vi "Coordinate Space_Setting_UI.vi"(9 "RootPath":path, 10 "Project Name":string, 11 "Image In":T1(plugin-control)) -> (3 "Origin Set":bool)   [LabVIEW 2019]
uses:
  Control/CoordinateUI.ctl
  Control/CoordinateAction.ctl
  Control/DataTransform.ctl
  Process/Controls/Process_Setting.ctl
  Analysis/Controls/Analysis_Setting.ctl
  Controls/Vision_DataEntry.ctl
  Caliper/Controls/Caliper_Entry_FGV_Action.ctl
  Caliper/Controls/AnalysisResultPointsAction.ctl
  Caliper/Controls/CaliperType.ctl
  Caliper/Controls/SelectionListEntryPointType.ctl
  Caliper/Controls/SelectionListEntry.ctl
  Control/CoordinateCaliperSetting.ctl
  Caliper/Controls/CaliperResult.ctl
  Caliper/Controls/CaliperDataEntry.ctl
  <vilib>/Utility/miscctls.llb/LVRowAndColumnTypeDef.ctl
  Analysis/Controls/V_Analysis_Type.ctl
  Ctrl/VisionProcessName.ctl
  Control/CoordinateAnalysisFunc.ctl
panel:
  in  "Done":bool
  out "Numeric":i32
  out "x-y":u32
  out "TempImage":T1(plugin-control)
  in  "Available Points":i32(listbox)=5
  in  "Function_Tab":enum32{"Process", "Analysis", "Caliper"}(tab)
  out "Process Steps":i32(listbox)
  in  "ConfigProcess":bool
  in  "ConfigAnalysis Modify":bool caption="Modify"
  in  "Analysis Delete":bool caption="Delete"
  in  "Analysis Step":i32[](listbox)
  in  "ConfigAnalysis":bool
  in  "Analysis Function":T2
  in  "Caliper Step":i32[](listbox)
  in  "Set Caliper":bool
  in  "Run Test":bool
  in  "CoordExit":bool caption="Exit"
  in  "Set Original":bool
  out "Vision_Image":T1(plugin-control)
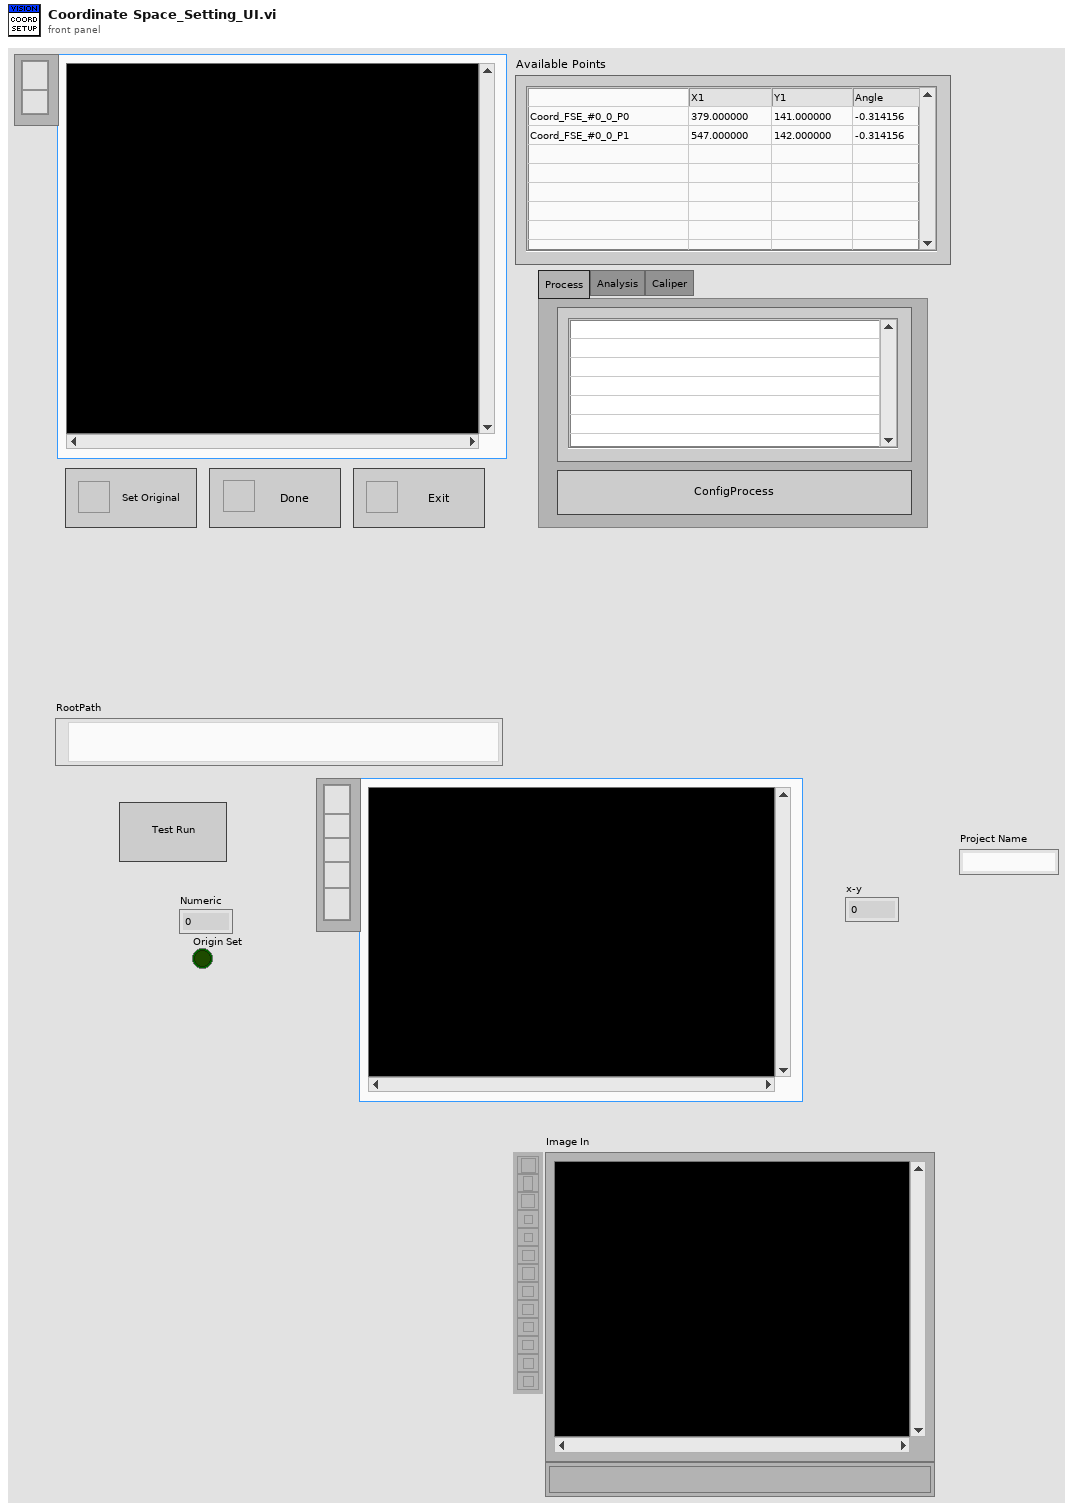
[diagram p1: front panel]
types:
  T1 = typedef "IMAQ Image.ctl" = refnum<image>
  T2 = typedef "CoordinateAnalysisFunc.ctl" = enum16{"Pattern Match", "Find Straight Edge"}
  T3 = typedef "CoordinateUI.ctl" = cluster{"CoordinateUICmd":enum16{"Initialize", "ConfigProcess", "AddAnalysis", "EditAnalysis", "SingleRunWithoutCaliper", "UpdateCaliper", "Run Test", "DeleteAnalysis", "SetOrigin", "UIUpdate", "Done", "Stop", "OriginUpdate", "UpdateOriginList", "Init Read Template"}, "CoordiUIParam":variant}
  T4 = typedef "Image Type" = u32
  T5 = typedef "CoordinateAction.ctl" = enum16{"Initialize", "CoordEntryInput", "CoordEntryOutput", "CoordEntryTemp", "CoordEntryBackup", "CoordEntryReturn"}
  T6 = typedef "LVRowAndColumnTypeDef.ctl" = cluster{"Row":i32, "Column":i32}
  T7 = typedef "Caliper_Entry_FGV_Action.ctl" = enum16{"Init", "Close", "Add", "Delete", "ReplaceAll", "ReadAll"}
  T8 = typedef "Vision_DataEntry.ctl" = cluster{"vROIName":string, "vROIContour":cluster{"Contour Type":u32, "ROI Type":u32, "Points":i32[]}, "ProcessSetting":T9[], "Analysis_Setting":T11}
  T9 = typedef "Process_Setting.ctl" = cluster{"Enum_PreProcess":T10, "Parameter":string}
  T10 = typedef "VisionProcessName.ctl" = enum16{"*CamParameter*", "CamAttributes", "*Preprocess*", "CG_Brightness", "C_Plane Extraction", "C_Threshold", "G_Lookup Table", "G_Threshold"}
  T11 = typedef "Analysis_Setting.ctl" = cluster{"PreProcess":T12, "Parameter":string}
  T12 = typedef "V_Analysis_Type.ctl" = enum16{"None", "C_Color Pattern Matching", "G_PatternMatching", "G_ShapeDectect", "G_GeometricMatch", "B_Area Check"}
  T13 = typedef "DataTransform.ctl" = enum16{"CoordToMain", "MainToCoord"}
  T14 = typedef "CoordinateCaliperSetting.ctl" = cluster{"Result":variant, "CoordinateUse":bool, "CaliperEntry":T15}
  T15 = typedef "CaliperDataEntry.ctl" = cluster{"CaliperType":T16, "Points":T17[], "Result":T19, "StepName":string}
  T16 = typedef "CaliperType.ctl" = u32
  T17 = typedef "SelectionListEntry.ctl" = cluster{"Type":T18, "Index":i32}
  T18 = typedef "SelectionListEntryPointType.ctl" = enum16{"AnalysisResult", "CaliperResult"}
  T19 = typedef "CaliperResult.ctl" = cluster{"PointInclude?":bool, "Num_Of_Pts":u8, "Position.X":dbl, "Position.Y":dbl, "Angle":dbl, "Distance":dbl, "Area":dbl, "Radius_MAX":dbl, "Radius2_min":dbl, "Dev_Residual":dbl, "P2.X":dbl, "P2.Y":dbl, "StepName":string, "Point ID":u8, "StepError?":bool, "ResultDiff?":bool}
  T20 = typedef "AnalysisResultPointsAction.ctl" = enum16{"Init", "Add", "Delete", "ReplaceAll", "ReadAll", "Close"}
  T21 = enum16{"Initialize", "ConfigProcess", "AddAnalysis", "EditAnalysis", "SingleRunWithoutCaliper", "UpdateCaliper", "Run Test", "DeleteAnalysis", "SetOrigin", "UIUpdate", "Done", "Stop", "OriginUpdate", "UpdateOriginList", "Init Read Template"}
  T22 = typedef "CoordinatteEntry.ctl" = cluster{"ProcessSetting":T9[], "Project Name":string, "AnalysisSetting":T23[], "Coord?":bool, "OriginPointInfo":cluster{"Output Original":bool, "Origin Name":string, "Angle":dbl, "Mode":u16, "OriginPoint":cluster{"X":dbl, "Y":dbl}}, "CaliperSetting":T14[], "CoordIndex":i32[]}
  T23 = typedef "CoordinateAnalysisSetting.ctl" = cluster{"Analysis_Type":enum16{"PatternMatch", "Straight Edge"}, "ROI ":T24, "Parameter":variant, "Step Result":variant, "AnalysisStepName":string, "CoordinateUse":bool}
  T24 = typedef "ROI Descriptor" = cluster{"Global Rectangle":i32[], "Contours":cluster{"ID":enum32{"External", "Internal"}, "Type":u32, "Coordinates":i32[]}[]}
  T25 = typedef "Analysis_Setting.ctl" = cluster{"PreProcess":T26, "Parameter":string}
  T26 = typedef "V_Analysis_Type.ctl" = enum16{"None", "C_Color Pattern Matching", "G_PatternMatching"}
  T27 = typedef "Analysis_Setting.ctl" = cluster{"PreProcess":T28, "Parameter":string}
  T28 = typedef "VisionProcessName.ctl" = enum16{"*CamParameter*", "CamAttributes", "*Preprocess*", "CG_Brightness", "C_Plane Extraction", "C_Threshold", "G_Lookup Table", "G_Threshold", "B_Image Inversion", "*Algorithm*", "CG_Histogram", "C_Color Matching", "C_Color Pattern Matching", "G_PatternMatch", "CG_Find Straight Edge", "CG_Adv. Find Straight Edge", "CG_Find Circular Edge", "G_Max Clamp", "G_Clamp (Rake)", "G_Pattern Matching"}
  T29 = typedef "Analysis_Result_To_Caliper.ctl" = cluster{"PointName":string, "Position_X":dbl, "Position_Y":dbl}
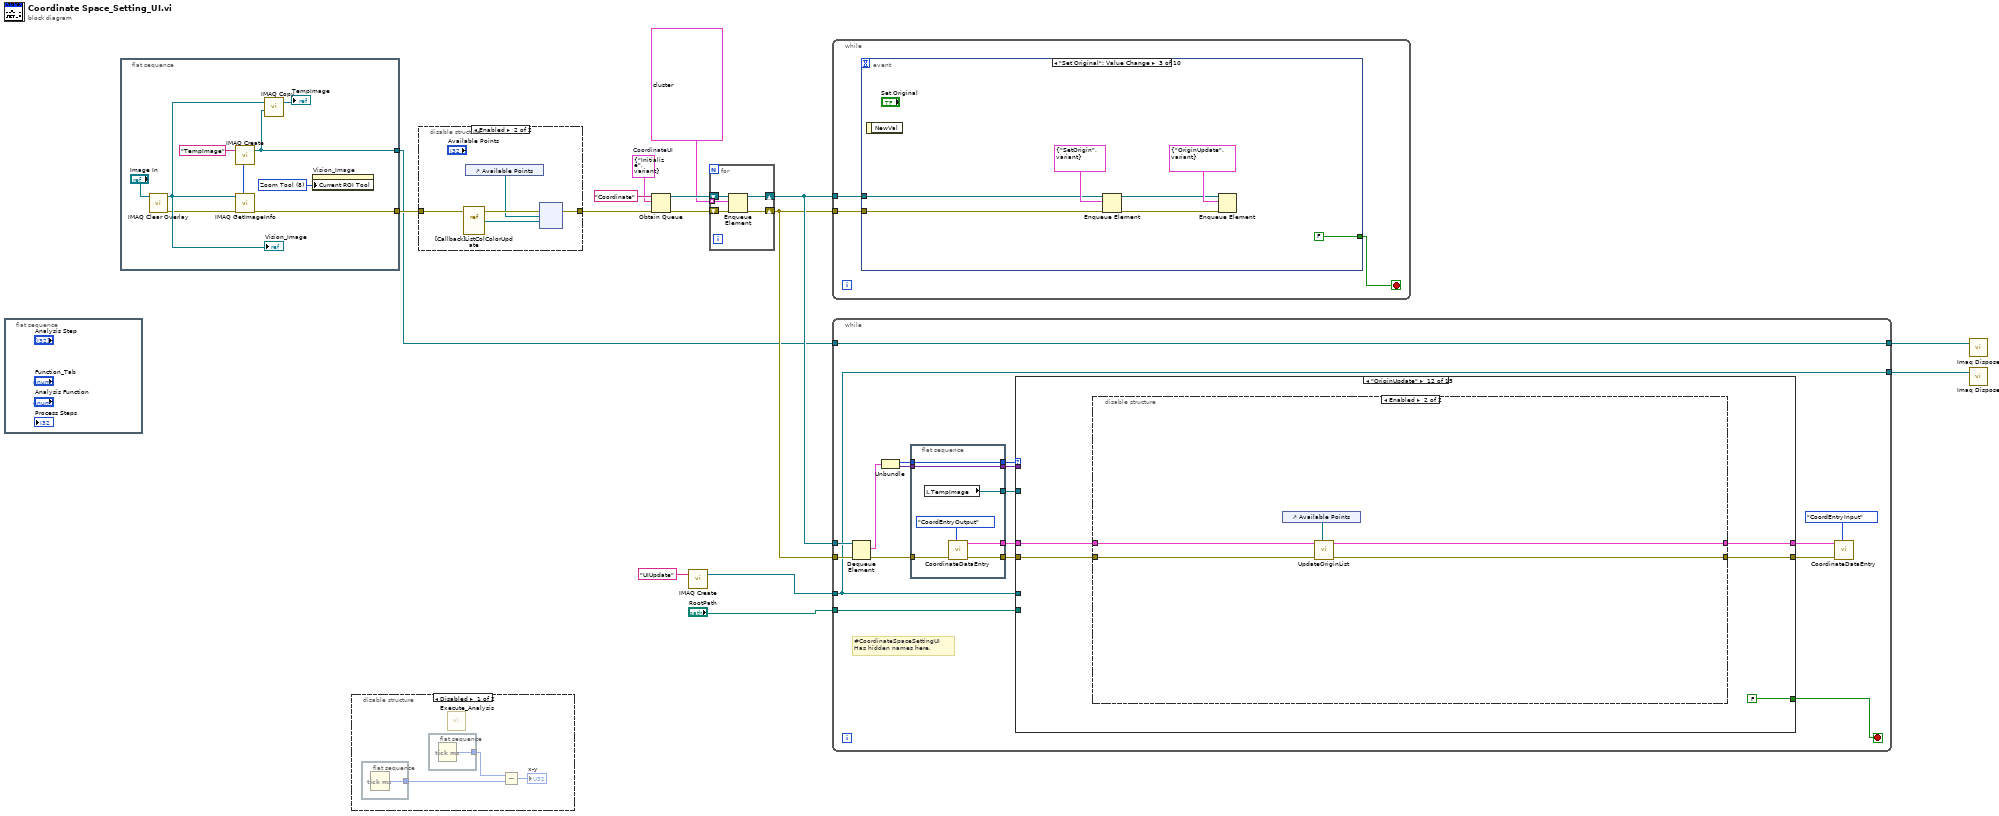
[diagram p0: block diagram]
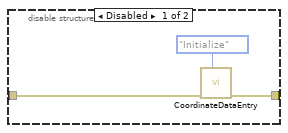
[diagram p2: hidden frame]
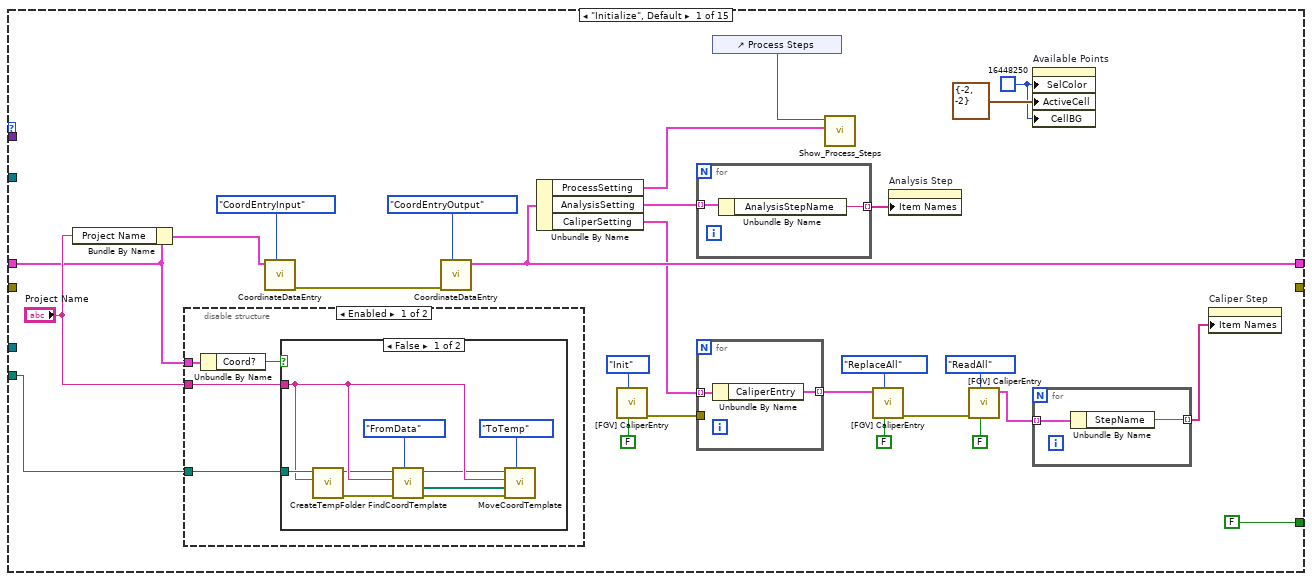
[diagram p4: hidden frame]
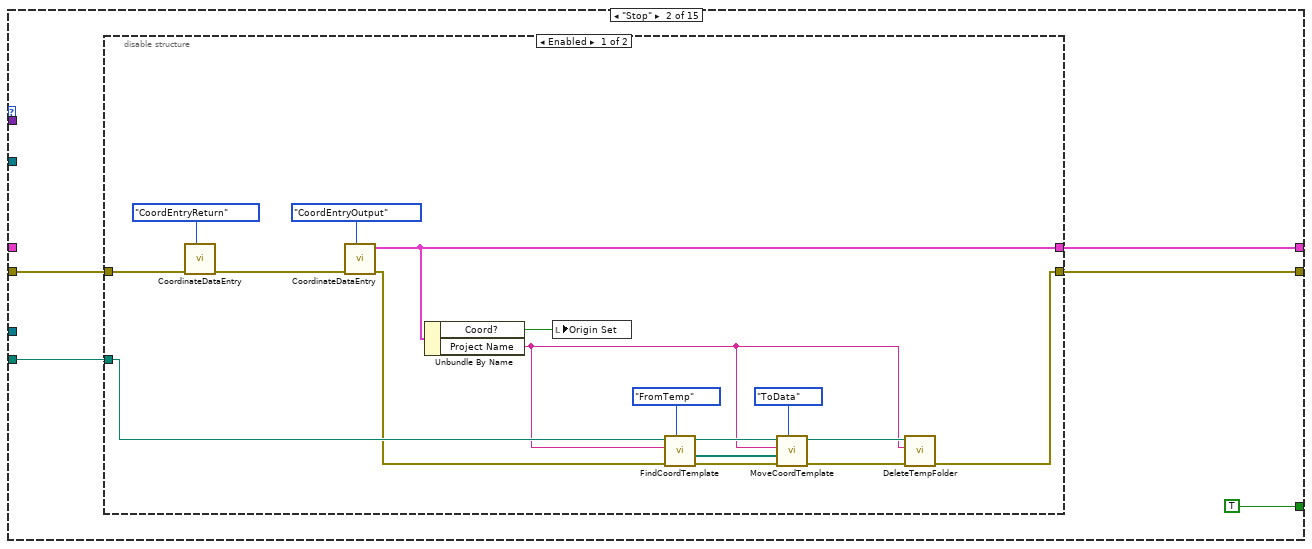
[diagram p7: hidden frame]
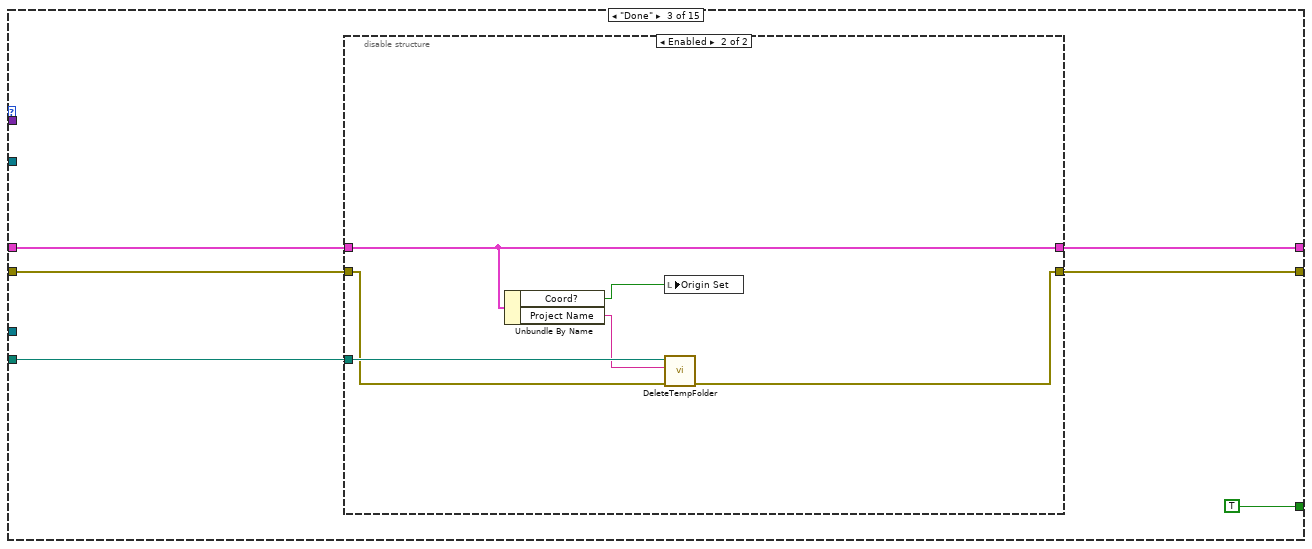
[diagram p9: hidden frame]
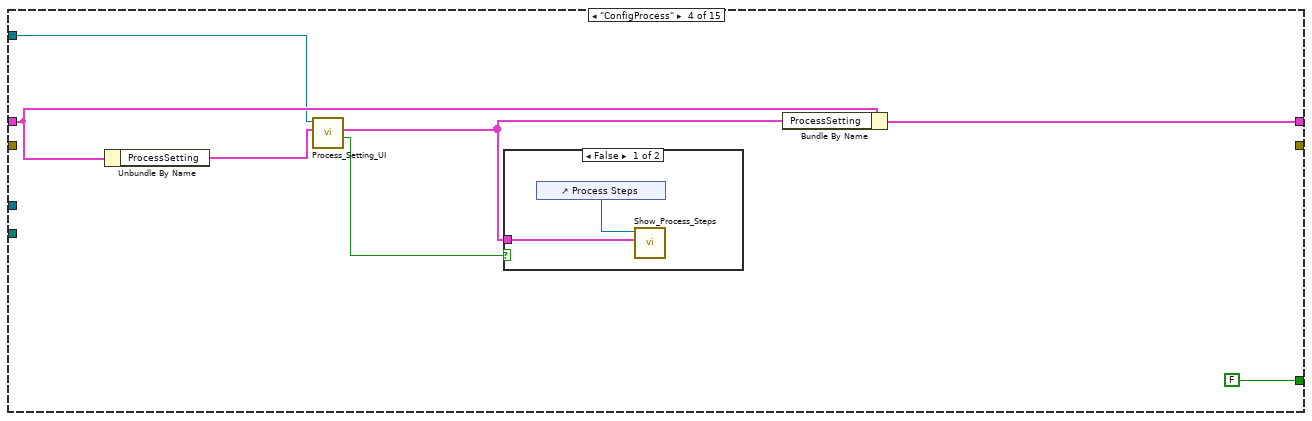
[diagram p11: hidden frame]
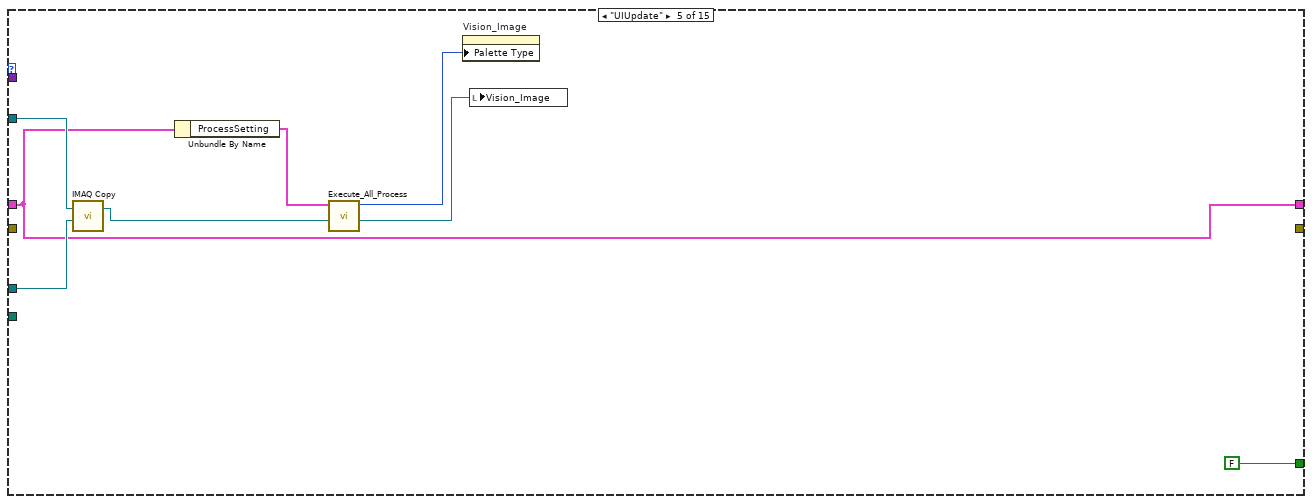
[diagram p13: hidden frame]
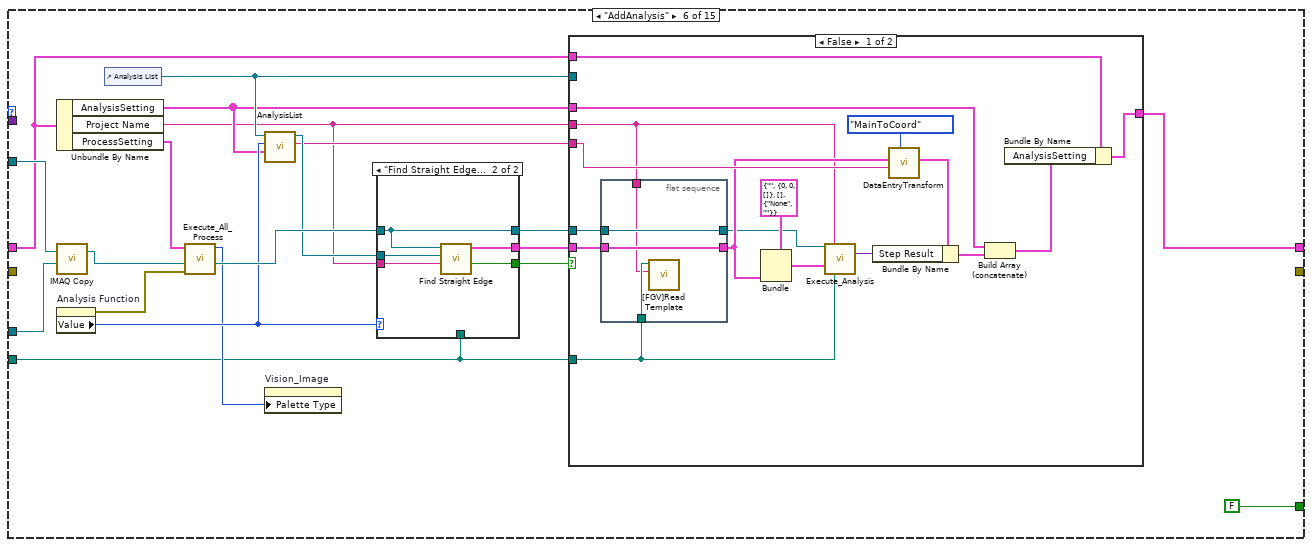
[diagram p14: hidden frame]
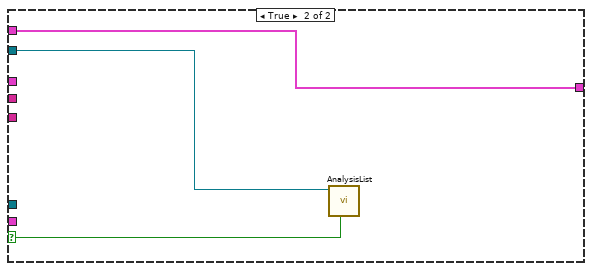
[diagram p15: hidden frame]
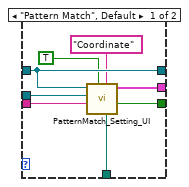
[diagram p16: hidden frame]
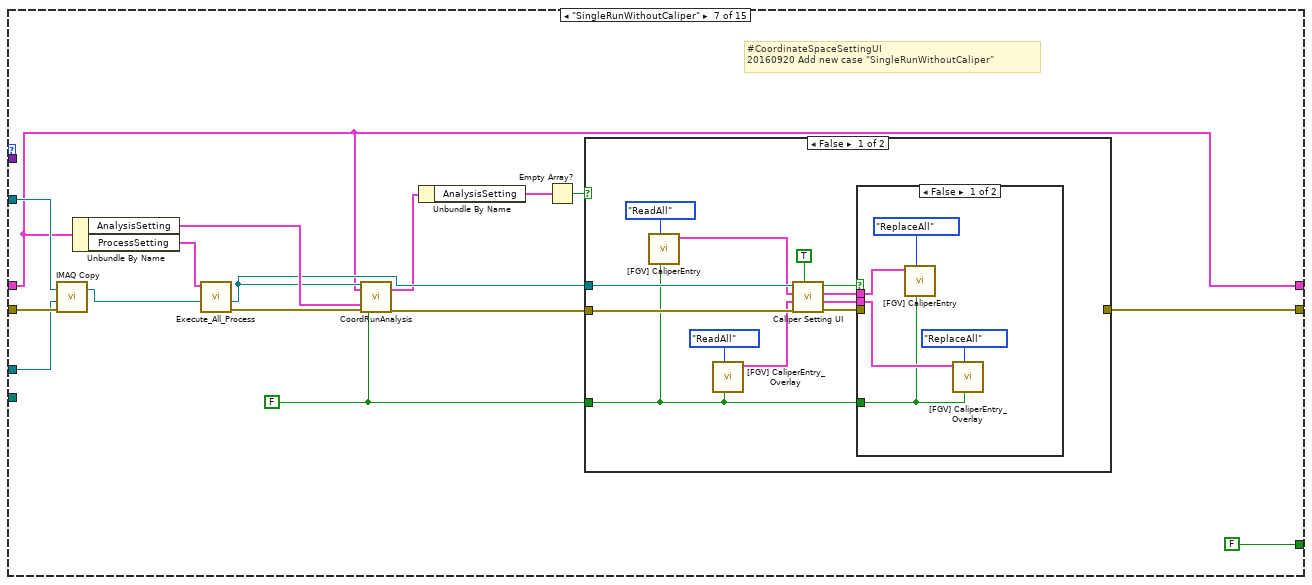
[diagram p17: hidden frame]
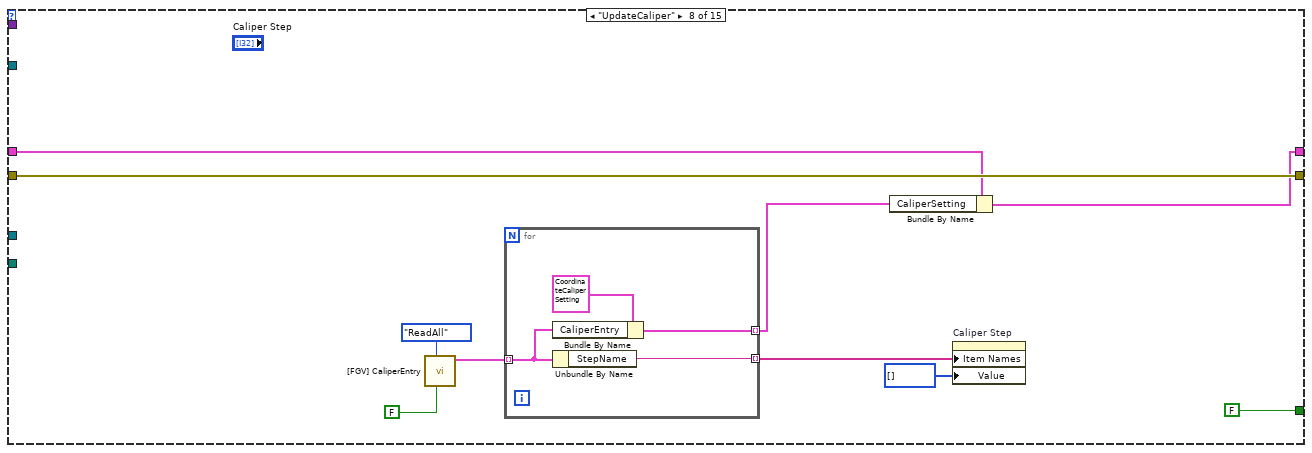
[diagram p20: hidden frame]
diagram:
  w14 = T3 {"CoordinateUICmd"=enum."Initialize", "CoordiUIParam"=variant}  # CoordinateUI
  n1 = flat-sequence {
    frame #0 {
    }
  }
  n2 = flat-sequence {
    tunnel: [w22] -> w6
    tunnel: [w19] -> w2
    frame #0 {
      w16 = u32 8 items=["Zoom Tool"=8, "Selection Tool"=0, "Pan Tool"=9, "Point Tool"=1, "Line Tool"=2, "Rectangle Tool"=3, "Rotated Rectangle Tool"=12, "Polyline Tool"=10, "Polygon Tool"=5, "Freehand Tool"=11, "Closed Freehand Tool"=6, "Ellipse Tool"=4, "Annulus Tool"=7] ("Current ROI Tool")
      n3 = call "IMAQ Clear Overlay"("Image"="Image In") -> ("error out"=w18:errorcluster, "Image Out"=w21:T1)  [unwired: 9 in]
      "Vision_Image" <- w21
      n4 = call "IMAQ GetImageInfo"("error in (no error)"=w18, "Image"=w21) -> ("error out"=w22:errorcluster, "Image Type"=w20:T4)  [unwired: 2 in, 6 out]
      n5 = call "IMAQ Create"("Image Name"="TempImage", "Image Type"=w20) -> ("New Image"=w19:T1)  [unwired: 3 in, 1 out]
      n6 = call "IMAQ Copy"("Image Dst"=w19, "Image Src"=w21) -> ("Image Dst Out"=→"TempImage":T1)  [unwired: 4 in, 1 out]
      n7 = property on="Vision_Image" class="ImageControl"("Current ROI Tool"=w16) -> ()  [unwired: 2 in, 2 out]
    }
  }
  n8 = disable-structure shown="Disabled" {
    frame Disabled {
      n9 = flat-sequence {
        tunnel: [w29] -> w26
        frame #0 {
          n10 = Tick Count (ms)() -> (millisecond timer value=w29:u32)
        }
      }
      n11 = flat-sequence {
        tunnel: [w28] -> w25
        frame #0 {
          n12 = Tick Count (ms)() -> (millisecond timer value=w28:u32)
        }
      }
      n13 = call "Execute_Analysis.vi"() -> ()  [unwired: 8 in, 4 out]
      n14 = Subtract(x=w25, y=w26) -> (x-y=→"x-y":u32)
    }
    frame Enabled {
    }
  }
  n15 = disable-structure shown="Enabled" {
    disable-tunnel: [w32 w34] -> w9
    disable-tunnel: w6 -> [w31 w36]
    frame Disabled {
      n16 = call "CoordinateDataEntry.vi"("CoordinateAction"=CoordinateAction."Initialize", "error in (no error)"=w31) -> ("error out"=w32:errorcluster)  [unwired: 8 in, 1 out]
    }
    frame Enabled {
      n17 = vi-ref "[Callback]ListColColorUpdate.vi"() -> ("vi reference"=w33:refnum<vi>)
      n18 = control-ref of="Available Points"() -> (w35:refnum<vi>)
      n19 = node(w36, w35, w33) -> (w34:errorcluster)  [unwired: 2 in, 1 out]
    }
  }
  n20 = Obtain Queue(name (unnamed)="Coordinate", element data type=w14, error in (no error)=w9) -> (queue out=w13:refnum<queue>, error out=w12:errorcluster)  [unwired: 2 in, 1 out]
  n21 = call "IMAQ Create"("Image Name"="UIUpdate") -> ("New Image"=w7:T1)  [unwired: 4 in, 1 out]
  n22 = for {
    shift-right: [w39] -> w11
    shift-left: w13 -> [w41]
    shift-right: [w38] -> w10
    shift-left: w12 -> [w40]
    tunnel: T3[] [{"CoordinateUICmd"=enum."Initialize", "CoordiUIParam"=variant}, {"CoordinateUICmd"=enum."Init Read Template", "CoordiUIParam"=variant}, {"CoordinateUICmd"=enum."Run Test", "CoordiUIParam"=variant}, {"CoordinateUICmd"=enum."OriginUpdate", "CoordiUIParam"=variant}] -> [w37] mode=indexing
    n23 = Enqueue Element(queue=w41, element=w37, error in (no error)=w40) -> (queue out=w39:refnum<queue>, error out=w38:errorcluster)  [unwired: 1 in, 1 out]
  }
  n24 = while {
    tunnel: w10 -> [w44]
    tunnel: w11 -> [w43]
    stop <- w42 stop-if-true
    n25 = event shown="[2] \"Set Original\": Value Change" {
      selector: _ -> [_ _ _ _ _ _ _ _ _ _]
      dyn-events: _ -> [_ _ _ _ _ _ _ _ _ _]
      timeout: _ -> [_ _ _ _ _ _ _ _ _ _]
      tunnel: w44 -> [w47 w49 w56 w65 w78 w90 w94 w117 w127 w131]
      tunnel: w43 -> [w48 w50 w57 w66 w79 w91 w95 w118 w128 w132]
      tunnel: [TRUE ("Cancel") TRUE ("Cancel") FALSE ("Cancel") FALSE ("Cancel") FALSE ("Cancel") FALSE ("Cancel") FALSE ("Cancel") FALSE ("Cancel") FALSE ("Cancel") FALSE ("Cancel")] -> w42
      event "CoordExit": Value Change {
        n26 = event-data() -> ()  [unwired: 1 in, 1 out]
        n27 = Enqueue Element(queue=w48, element=T3 {"CoordinateUICmd"=enum."Stop", "CoordiUIParam"=variant}, error in (no error)=w47) -> ()  [unwired: 1 in, 3 out]
      }
      event "Done": Value Change {
        n28 = event-data() -> ()  [unwired: 1 in, 1 out]
        n29 = Enqueue Element(queue=w50, element=T3 {"CoordinateUICmd"=enum."Done", "CoordiUIParam"=variant}, error in (no error)=w49) -> ()  [unwired: 1 in, 3 out]
      }
      event "Set Original": Value Change {
        n30 = event-data() -> ()  [unwired: 1 in, 1 out]
        n31 = Enqueue Element(queue=w57, element=T3 {"CoordinateUICmd"=enum."SetOrigin", "CoordiUIParam"=variant}, error in (no error)=w56) -> (queue out=w53:refnum<queue>, error out=w54:errorcluster)  [unwired: 1 in, 1 out]
        n32 = Enqueue Element(queue=w53, element=T3 {"CoordinateUICmd"=enum."OriginUpdate", "CoordiUIParam"=variant}, error in (no error)=w54) -> ()  [unwired: 1 in, 3 out]
      }
      event "ConfigProcess": Value Change {
        n33 = event-data() -> ()  [unwired: 1 in, 1 out]
        n34 = Enqueue Element(queue=w66, element=T3 {"CoordinateUICmd"=enum."ConfigProcess", "CoordiUIParam"=variant}, error in (no error)=w65) -> (queue out=w62:refnum<queue>, error out=w63:errorcluster)  [unwired: 1 in, 1 out]
        n35 = Enqueue Element(queue=w62, element=T3 {"CoordinateUICmd"=enum."UIUpdate", "CoordiUIParam"=variant}, error in (no error)=w63) -> ()  [unwired: 1 in, 3 out]
      }
      event "ConfigAnalysis": Value Change {
        n36 = event-data() -> ()  [unwired: 1 in, 1 out]
        n37 = Enqueue Element(queue=w79, element=T3 {"CoordinateUICmd"=enum."AddAnalysis", "CoordiUIParam"=variant}, error in (no error)=w78) -> (queue out=w76:refnum<queue>, error out=w77:errorcluster)  [unwired: 1 in, 1 out]
        n38 = Enqueue Element(queue=w76, element=T3 {"CoordinateUICmd"=enum."UIUpdate", "CoordiUIParam"=variant}, error in (no error)=w77) -> (queue out=w72:refnum<queue>, error out=w73:errorcluster)  [unwired: 1 in, 1 out]
        n39 = Enqueue Element(queue=w72, element=T3 {"CoordinateUICmd"=enum."Run Test", "CoordiUIParam"=variant}, error in (no error)=w73) -> (queue out=w68:refnum<queue>, error out=w67:errorcluster)  [unwired: 1 in, 1 out]
        n40 = Enqueue Element(queue=w68, element=T3 {"CoordinateUICmd"=enum."OriginUpdate", "CoordiUIParam"=variant}, error in (no error)=w67) -> ()  [unwired: 1 in, 3 out]
      }
      event "Set Caliper": Value Change {
        n41 = event-data() -> ()  [unwired: 1 in, 1 out]
        n42 = Enqueue Element(queue=w91, element=T3 {"CoordinateUICmd"=enum."SingleRunWithoutCaliper", "CoordiUIParam"=variant}, error in (no error)=w90) -> (queue out=w87:refnum<queue>, error out=w86:errorcluster)  [unwired: 1 in, 1 out]
        n43 = Enqueue Element(queue=w87, element=T3 {"CoordinateUICmd"=enum."UpdateCaliper", "CoordiUIParam"=variant}, error in (no error)=w86) -> (queue out=w85:refnum<queue>, error out=w84:errorcluster)  [unwired: 1 in, 1 out]
        n44 = Enqueue Element(queue=w85, element=T3 {"CoordinateUICmd"=enum."Run Test", "CoordiUIParam"=variant}, error in (no error)=w84) -> (queue out=w81:refnum<queue>, error out=w80:errorcluster)  [unwired: 1 in, 1 out]
        n45 = Enqueue Element(queue=w81, element=T3 {"CoordinateUICmd"=enum."OriginUpdate", "CoordiUIParam"=variant}, error in (no error)=w80) -> ()  [unwired: 1 in, 3 out]
      }
      event "Analysis Step": Mouse Down {
        n46 = event-data() -> ("Mods.Double Click"=w96:bool)  [unwired: 1 in]
        n47 = case shown="False" w96 {
          tunnel: w95 -> [_ w105]
          tunnel: w94 -> [_ w104]
          frame False {
          }
          frame True {
            n48 = Enqueue Element(queue=w105, element=T3 {"CoordinateUICmd"=enum."EditAnalysis", "CoordiUIParam"=variant}, error in (no error)=w104) -> (queue out=w107:refnum<queue>, error out=w108:errorcluster)  [unwired: 1 in, 1 out]
            n49 = Enqueue Element(queue=w107, element=T3 {"CoordinateUICmd"=enum."UIUpdate", "CoordiUIParam"=variant}, error in (no error)=w108) -> (queue out=w101:refnum<queue>, error out=w102:errorcluster)  [unwired: 1 in, 1 out]
            n50 = Enqueue Element(queue=w101, element=T3 {"CoordinateUICmd"=enum."Run Test", "CoordiUIParam"=variant}, error in (no error)=w102) -> (queue out=w98:refnum<queue>, error out=w97:errorcluster)  [unwired: 1 in, 1 out]
            n51 = Enqueue Element(queue=w98, element=T3 {"CoordinateUICmd"=enum."OriginUpdate", "CoordiUIParam"=variant}, error in (no error)=w97) -> ()  [unwired: 1 in, 3 out]
          }
        }
      }
      event "ConfigAnalysis Modify": Value Change {
        n52 = event-data() -> ()  [unwired: 1 in, 1 out]
        n53 = Enqueue Element(queue=w118, element=T3 {"CoordinateUICmd"=enum."EditAnalysis", "CoordiUIParam"=variant}, error in (no error)=w117) -> (queue out=w115:refnum<queue>, error out=w116:errorcluster)  [unwired: 1 in, 1 out]
        n54 = Enqueue Element(queue=w115, element=T3 {"CoordinateUICmd"=enum."UIUpdate", "CoordiUIParam"=variant}, error in (no error)=w116) -> (queue out=w112:refnum<queue>, error out=w111:errorcluster)  [unwired: 1 in, 1 out]
        n55 = Enqueue Element(queue=w112, element=T3 {"CoordinateUICmd"=enum."Run Test", "CoordiUIParam"=variant}, error in (no error)=w111) -> ()  [unwired: 1 in, 3 out]
      }
      event "Analysis Delete": Value Change {
        n56 = event-data() -> ()  [unwired: 1 in, 1 out]
        n57 = Enqueue Element(queue=w128, element=T3 {"CoordinateUICmd"=enum."DeleteAnalysis", "CoordiUIParam"=variant}, error in (no error)=w127) -> (queue out=w124:refnum<queue>, error out=w123:errorcluster)  [unwired: 1 in, 1 out]
        n58 = Enqueue Element(queue=w124, element=T3 {"CoordinateUICmd"=enum."Run Test", "CoordiUIParam"=variant}, error in (no error)=w123) -> (queue out=w120:refnum<queue>, error out=w119:errorcluster)  [unwired: 1 in, 1 out]
        n59 = Enqueue Element(queue=w120, element=T3 {"CoordinateUICmd"=enum."OriginUpdate", "CoordiUIParam"=variant}, error in (no error)=w119) -> ()  [unwired: 1 in, 3 out]
      }
      event "Run Test": Value Change {
        n60 = event-data() -> ()  [unwired: 1 in, 1 out]
        n61 = Enqueue Element(queue=w132, element=T3 {"CoordinateUICmd"=enum."Run Test", "CoordiUIParam"=variant}, error in (no error)=w131) -> ()  [unwired: 1 in, 3 out]
      }
    }
  }
  n62 = while {
    tunnel: w11 -> [w150]
    tunnel: w10 -> [w149]
    tunnel: w7 -> [w141]
    tunnel: [w141] -> w4
    tunnel: [w140] -> w3
    tunnel: w2 -> [w140]
    tunnel: "RootPath" -> [w139]
    stop <- w135 stop-if-true
    # "#CoordinateSpaceSettingUI\nHas hidden names here."
    n63 = Dequeue Element(queue=w150, error in (no error)=w149) -> (element=w148:T3, error out=w147:errorcluster)  [unwired: 1 in, 2 out]
    n64 = Unbundle(w148) -> ("CoordinateUICmd"=w136:T21, "CoordiUIParam"=w134:variant)
    n65 = flat-sequence {
      tunnel: w147 -> [w157]
      tunnel: [w156] -> w146
      tunnel: [w155] -> w145
      tunnel: [w154] -> w144
      tunnel: [w152] -> w137
      tunnel: w136 -> [w152]
      tunnel: w134 -> [w151]
      tunnel: [w151] -> w133
      frame #0 {
        n66 = local read "TempImage"() -> (w154:T1)
        n67 = call "CoordinateDataEntry.vi"("CoordinateAction"=CoordinateAction."CoordEntryOutput", "error in (no error)"=w157) -> ("error out"=w155:errorcluster, "CoordinatteEntry Output"=w156:T22)  [unwired: 8 in]
      }
    }
    n68 = case shown="\"OriginUpdate\"" w137 {
      tunnel: [FALSE ("Cancel") TRUE ("Cancel") TRUE ("Cancel") FALSE ("Cancel") FALSE ("Cancel") FALSE ("Cancel") FALSE ("Cancel") FALSE ("Cancel") FALSE ("Cancel") FALSE ("Cancel") FALSE ("Cancel") FALSE ("Cancel") FALSE ("Cancel") FALSE ("Cancel") FALSE ("Cancel")] -> w135
      tunnel: w146 -> [w160 _ w229 w245 w249 w271 w318 w350 w393 w426 w442 w478 w518 w565 w568]
      tunnel: w145 -> [_ w207 w231 _ _ _ w323 w351 _ w430 w439 w476 _ w561 _]
      tunnel: w144 -> [_ _ _ w241 w253 w275 w324 _ w400 w434 _ _ w525 _ _]
      tunnel: w141 -> [_ _ _ _ w252 w274 w322 _ w399 _ _ _ w508 _ _]
      tunnel: [w176 w205 w228 w240 w249 w263 w318 w349 w392 w426 w441 w474 w513 w564 w568] -> w142
      tunnel: w139 -> [w162 w204 w227 _ _ w259 _ _ w390 _ _ _ w506 _ w570]
      tunnel: [_ w206 w230 _ _ _ w319 w351 w389 w427 w438 w475 _ w560 w569] -> w138
      tunnel: w133 -> [_ _ _ _ _ _ _ _ _ w432 _ _ _ _ _]
      frame "Initialize", Default {
        w158 = u32 16448250
        n69 = Bundle By Name(cluster=w160, "Project Name"="Project Name") -> (w184:T22)
        n70 = disable-structure shown="Enabled" {
          disable-tunnel: w162 -> [w188 _]
          disable-tunnel: "Project Name" -> [w187 _]
          disable-tunnel: w160 -> [w186 _]
          frame Enabled {
            n71 = Unbundle By Name(w186) -> ("Coord?"=w185:bool)
            n72 = case shown="False" w185 {
              tunnel: w188 -> [w197 _]
              tunnel: w187 -> [w196 _]
              frame False {
                n73 = call "CreateTempFolder.vi"("Project"=w196, "Root In"=w197) -> ("error out"=w195:errorcluster, "Root Out"=w193:path)  [unwired: 8 in]
                n74 = call "FindCoordTemplate.vi"("FindAction"=enum16{"FromTemp", "FromData"}."FromData", "error in (no error)"=w195, "Project"=w196, "Root In"=w193) -> ("error out"=w194:errorcluster, "CoordTemplatePaths"=w191:path[], "Root Out"=w192:path)  [unwired: 5 in]
                n75 = call "MoveCoordTemplate.vi"("MoveAction"=enum16{"ToTemp", "ToData"}."ToTemp", "error in (no error)"=w194, "Paths"=w191, "Project"=w196, "Root In"=w192) -> ()  [unwired: 5 in, 2 out]
              }
              frame True {
              }
            }
          }
          frame Disabled {
          }
        }
        n76 = call "CoordinateDataEntry.vi"("CoordinateAction"=CoordinateAction."CoordEntryInput", "OneCoordStep Input"=w184) -> ("error out"=w182:errorcluster)  [unwired: 8 in, 1 out]
        n77 = call "CoordinateDataEntry.vi"("CoordinateAction"=CoordinateAction."CoordEntryOutput", "error in (no error)"=w182) -> ("CoordinatteEntry Output"=w176:T22)  [unwired: 8 in, 1 out]
        n78 = Unbundle By Name(w176) -> ("ProcessSetting"=w180:T9[], "AnalysisSetting"=w178:T23[], "CaliperSetting"=w169:T14[])
        n79 = call "[FGV] CaliperEntry.vi"("CoordSystemRun"=FALSE, "Action"=Caliper_Entry_FGV_Action."Init") -> ("error out"=w164:errorcluster)  [unwired: 8 in, 1 out]
        n80 = for {
          tunnel: w178 -> [w203] mode=indexing
          tunnel: [w202] -> w177 mode=indexing
          n81 = Unbundle By Name(w203) -> ("AnalysisStepName"=w202:string)
        }
        n82 = for {
          tunnel: w169 -> [w199] mode=indexing
          tunnel: [w198] -> w168 mode=indexing
          tunnel: w164 -> [_]
          n83 = Unbundle By Name(w199) -> ("CaliperEntry"=w198:T15)
        }
        n84 = control-ref of="Process Steps"() -> (w179:refnum<vi>)
        n85 = call "Show_Process_Steps.vi"("ProcessSettingIn"=w180, "ProcessSteps"=w179) -> ()  [unwired: 9 in, 1 out]
        n86 = call "[FGV] CaliperEntry.vi"("CoordSystemRun"=FALSE, "Action"=Caliper_Entry_FGV_Action."ReplaceAll", "CaliperEntriesIn"=w168) -> ("error out"=w167:errorcluster)  [unwired: 7 in, 1 out]
        n87 = property on="Analysis Step" class="LstBox (strict)"("Item Names"=w177) -> ()  [unwired: 2 in, 2 out]
        n88 = call "[FGV] CaliperEntry.vi"("CoordSystemRun"=FALSE, "Action"=Caliper_Entry_FGV_Action."ReadAll", "error in (no error)"=w167) -> ("AllCaliperEntries"=w174:T15[])  [unwired: 7 in, 1 out]
        n89 = property on="Available Points" class="MCListbox (strict)"("SelColor"=w158, "ActiveCell"=T6 {"Row"=-2, "Column"=-2} ("Active Cell:Active Cell"), "CellBG"=w158) -> ()  [unwired: 2 in, 2 out]
        n90 = for {
          tunnel: w174 -> [w201] mode=indexing
          tunnel: [w200] -> w172 mode=indexing
          n91 = Unbundle By Name(w201) -> ("StepName"=w200:string)
        }
        n92 = property on="Caliper Step" class="LstBox (strict)"("Item Names"=w172) -> ()  [unwired: 2 in, 2 out]
      }
      frame "Stop" {
        n93 = disable-structure shown="Enabled" {
          disable-tunnel: w207 -> [w222 w226]
          disable-tunnel: [w211 w226] -> w206
          disable-tunnel: [w210 _] -> w205
          disable-tunnel: w204 -> [w215 _]
          frame Enabled {
            n94 = call "CoordinateDataEntry.vi"("CoordinateAction"=CoordinateAction."CoordEntryReturn", "error in (no error)"=w222) -> ("error out"=w225:errorcluster)  [unwired: 8 in, 1 out]
            n95 = call "CoordinateDataEntry.vi"("CoordinateAction"=CoordinateAction."CoordEntryOutput", "error in (no error)"=w225) -> ("error out"=w212:errorcluster, "CoordinatteEntry Output"=w210:T22)  [unwired: 8 in]
            n96 = Unbundle By Name(w210) -> ("Coord?"=w221:bool, "Project Name"=w209:string)
            n97 = local write "Origin Set"(w221) -> ()
            n98 = call "FindCoordTemplate.vi"("FindAction"=enum16{"FromTemp", "FromData"}."FromTemp", "error in (no error)"=w212, "Project"=w209, "Root In"=w215) -> ("error out"=w220:errorcluster, "CoordTemplatePaths"=w218:path[], "Root Out"=w219:path)  [unwired: 5 in]
            n99 = call "MoveCoordTemplate.vi"("MoveAction"=enum16{"ToTemp", "ToData"}."ToData", "error in (no error)"=w220, "Paths"=w218, "Project"=w209, "Root In"=w219) -> ("error out"=w214:errorcluster, "Root Out"=w213:path)  [unwired: 5 in]
            n100 = call "DeleteTempFolder.vi"("error in (no error)"=w214, "Project"=w209, "Root"=w213) -> ("error out"=w211:errorcluster)  [unwired: 8 in]
          }
          frame Disabled {
          }
        }
      }
      frame "Done" {
        n101 = disable-structure shown="Enabled" {
          disable-tunnel: w231 -> [_ w237]
          disable-tunnel: [_ w235] -> w230
          disable-tunnel: w229 -> [_ w236]
          disable-tunnel: [_ w236] -> w228
          disable-tunnel: w227 -> [_ w238]
          frame Disabled {
          }
          frame Enabled {
            n102 = Unbundle By Name(w236) -> ("Coord?"=w233:bool, "Project Name"=w234:string)
            n103 = local write "Origin Set"(w233) -> ()
            n104 = call "DeleteTempFolder.vi"("error in (no error)"=w237, "Project"=w234, "Root"=w238) -> ("error out"=w235:errorcluster)  [unwired: 8 in]
          }
        }
      }
      frame "ConfigProcess" {
        n105 = Unbundle By Name(w245) -> ("ProcessSetting"=w244:T9[])
        n106 = call "Process_Setting_UI.vi"("ProcessSettingIn"=w244, "Vision_Image_In"=w241) -> ("Cancel?"=w243:bool, "ProcessSettingOut"=w242:T9[])  [unwired: 8 in]
        n107 = case shown="False" w243 {
          tunnel: w242 -> [w246 _]
          frame False {
            n108 = control-ref of="Process Steps"() -> (w247:refnum<vi>)
            n109 = call "Show_Process_Steps.vi"("ProcessSettingIn"=w246, "ProcessSteps"=w247) -> ()  [unwired: 9 in, 1 out]
          }
          frame True {
          }
        }
        n110 = Bundle By Name(cluster=w245, "ProcessSetting"=w242) -> (w240:T22)
      }
      frame "UIUpdate" {
        n111 = call "IMAQ Copy"("Image Dst"=w252, "Image Src"=w253) -> ("Image Dst Out"=w251:T1)  [unwired: 4 in, 1 out]
        n112 = Unbundle By Name(w249) -> ("ProcessSetting"=w254:T9[])
        n113 = call "Execute_All_Process.vi"("ImageIn"=w251, "ProcessSettingIn"=w254) -> ("Image Out"=w250:T1, "Palette Type"=w255:u32)  [unwired: 4 in, 4 out]
        n114 = property on="Vision_Image" class="ImageControl"("Palette Type"=w255) -> ()  [unwired: 2 in, 2 out]
        n115 = local write "Vision_Image"(w250) -> ()
      }
      frame "AddAnalysis" {
        n116 = Unbundle By Name(w271) -> ("AnalysisSetting"=w258:T23[], "Project Name"=w257:string, "ProcessSetting"=w270:T9[])
        n117 = call "IMAQ Copy"("Image Dst"=w274, "Image Src"=w275) -> ("Image Dst Out"=w273:T1)  [unwired: 4 in, 1 out]
        n118 = property on="Analysis Function" class="Enum (strict)"() -> (error out=w269:errorcluster, "Value"=w268:T2)  [unwired: 2 in, 1 out]
        n119 = control-ref of="Analysis List"() -> (w260:refnum<vi>)
        n120 = call "Execute_All_Process.vi"("error in (no error)"=w269, "ImageIn"=w273, "ProcessSettingIn"=w270) -> ("Image Out"=w272:T1, "Palette Type"=w262:u32)  [unwired: 3 in, 4 out]
        n121 = call "AnalysisList.vi"("AnalysisSetting"=w258, "Analysis Function"=w268, "Anallysis List in"=w260) -> ("AnalysisStpeName"=w266:string, "Anallysis List out"=w267:refnum<vi>)  [unwired: 6 in, 1 out]
        n122 = property on="Vision_Image" class="ImageControl"("Palette Type"=w262) -> ()  [unwired: 2 in, 2 out]
        n123 = case shown="\"Find Straight Edge\"" w268 {
          tunnel: [w307 w308] -> w261
          tunnel: [w306 w310] -> w264
          tunnel: w272 -> [w303 w309]
          tunnel: w267 -> [w305 w312]
          tunnel: w257 -> [w304 w311]
          tunnel: [w303 w309] -> w265
          tunnel: w259 -> [w301 _]
          frame "Pattern Match", Default {
            n124 = call "PatternMatch_Setting_UI.vi"("RootPath"=w301, "Type"="Coordinate", "Coord?"=TRUE, "ProjectName"=w304, "LstBox Refnum"=w305, "Vision_Image In"=w303) -> ("Cancel?"=w307:bool, "Analysis_Setting"=w306:T25)  [unwired: 3 in, 1 out]
          }
          frame "Find Straight Edge" {
            n125 = call "Find Straight Edge.vi"("ProjectName"=w311, "ROI List IN"=w312, "Vision_Image"=w309) -> ("Cancel?"=w308:bool, "Analysis_Setting"=w310:T27)  [unwired: 6 in, 1 out]
          }
        }
        n126 = case shown="False" w261 {
          selector: w261 -> [_ w297]
          tunnel: w271 -> [w292 w299]
          tunnel: [w291 w299] -> w263
          tunnel: w266 -> [w282 _]
          tunnel: w258 -> [w289 _]
          tunnel: w265 -> [w281 _]
          tunnel: w264 -> [w280 _]
          tunnel: w260 -> [_ w298]
          tunnel: w257 -> [w276 _]
          tunnel: w259 -> [w277 _]
          frame False {
            n127 = flat-sequence {
              tunnel: w281 -> [w296]
              tunnel: [w296] -> w278
              tunnel: w280 -> [w295]
              tunnel: [w295] -> w279
              tunnel: w277 -> [w294]
              tunnel: w276 -> [w293]
              frame #0 {
                n128 = call "[FGV]Read Template.vi"("Project Name"=w293, "RootPath"=w294) -> ()  [unwired: 9 in, 1 out]
              }
            }
            n129 = Bundle(cluster=T8 {"vROIName"="", "vROIContour"={"Contour Type"=0, "ROI Type"=0, "Points"=[]}, "ProcessSetting"=[], "Analysis_Setting"={"PreProcess"=enum."None", "Parameter"=""}} ("ROI Entry"), "Analysis_Setting"=w279) -> (w287:T8)  [unwired: 3 in]
            n130 = call "Execute_Analysis.vi"("Image In"=w278, "ProjectName"=w276, "ROI Entry"=w287, "RootPath"=w277) -> ("Result"=w285:variant)  [unwired: 7 in, 4 out]
            n131 = call "DataEntryTransform.vi"("DataTrasform"=DataTransform."MainToCoord", "AnalysisStepName"=w282, "MainSettingIn"=w279) -> ("CoordSettingOut"=w286:T23)  [unwired: 6 in, 2 out]
            n132 = Bundle By Name(cluster=w286, "Step Result"=w285) -> (w284:T23)
            n133 = Build Array (concatenate)(w289, w284) -> (w283:T23[])
            n134 = Bundle By Name(cluster=w292, "AnalysisSetting"=w283) -> (w291:T22)
          }
          frame True {
            n135 = call "AnalysisList.vi"("Cancel"=w297, "Anallysis List in"=w298) -> ()  [unwired: 7 in, 3 out]
          }
        }
      }
      frame "SingleRunWithoutCaliper" {
        w314 = FALSE ("CoordSystemRun?")
        # "#CoordinateSpaceSettingUI\n20160920 Add new case \"SingleRunWithoutCaliper\""
        n136 = call "IMAQ Copy"("error in (no error)"=w323, "Image Dst"=w322, "Image Src"=w324) -> ("Image Dst Out"=w328:T1)  [unwired: 3 in, 1 out]
        n137 = Unbundle By Name(w318) -> ("AnalysisSetting"=w325:T23[], "ProcessSetting"=w326:T9[])
        n138 = call "Execute_All_Process.vi"("ImageIn"=w328, "ProcessSettingIn"=w326) -> ("error out"=w327:errorcluster, "Image Out"=w320:T1)  [unwired: 4 in, 4 out]
        n139 = call "CoordRunAnalysis.vi"("Refnum in"=w320, "CoordinatteEntry In"=w318, "AnalysisSetting"=w325, "Error In"=w327, "CoordSystemRun?"=w314) -> ("CoordinatteEntry Out"=w317:T22, "Error Out"=w321:errorcluster)  [unwired: 11 in, 2 out]
        n140 = Unbundle By Name(w317) -> ("AnalysisSetting"=w316:T23[])
        n141 = Empty Array?(array=w316) -> (empty?=w315:bool)
        n142 = case shown="False" w315 {
          tunnel: w321 -> [w340 w346]
          tunnel: w320 -> [w339 _]
          tunnel: [_ w346] -> w319
          tunnel: w314 -> [w329 _]
          frame False {
            n143 = call "[FGV] CaliperEntry.vi"("CoordSystemRun"=w329, "Action"=Caliper_Entry_FGV_Action."ReadAll") -> ("AllCaliperEntries"=w335:T15[])  [unwired: 8 in, 1 out]
            n144 = call "[FGV] CaliperEntry_Overlay.vi"("CoordSystemRun"=w329, "Action"=Caliper_Entry_FGV_Action."ReadAll") -> ("AllCaliperEntries"=w336:T15[])  [unwired: 8 in, 1 out]
            n145 = call "Caliper Setting UI.vi"("Coor?"=TRUE, "error in (no error)"=w340, "CaliperEntryIn Overlay In"=w336, "CaliperEntryIn"=w335, "Vision_Image"=w339) -> ("error out"=w332:errorcluster, "CaliperEntryOut Overlay"=w330:T15[], "CaliperEntryOut"=w331:T15[], "Cancel?"=w333:bool)  [unwired: 3 in]
            n146 = case shown="False" w333 {
              tunnel: w332 -> [_ _]
              tunnel: w331 -> [w344 _]
              tunnel: w330 -> [w342 _]
              tunnel: w329 -> [w341 _]
              frame False {
                n147 = call "[FGV] CaliperEntry.vi"("CoordSystemRun"=w341, "Action"=Caliper_Entry_FGV_Action."ReplaceAll", "CaliperEntriesIn"=w344) -> ()  [unwired: 7 in, 2 out]
                n148 = call "[FGV] CaliperEntry_Overlay.vi"("CoordSystemRun"=w341, "Action"=Caliper_Entry_FGV_Action."ReplaceAll", "CaliperEntriesIn"=w342) -> ()  [unwired: 7 in, 2 out]
              }
              frame True {
              }
            }
          }
          frame True {
          }
        }
      }
      frame "UpdateCaliper" {
        n149 = call "[FGV] CaliperEntry.vi"("CoordSystemRun"=FALSE, "Action"=Caliper_Entry_FGV_Action."ReadAll") -> ("AllCaliperEntries"=w355:T15[])  [unwired: 8 in, 1 out]
        n150 = for {
          tunnel: w355 -> [w358] mode=indexing
          tunnel: [w360] -> w354 mode=indexing
          tunnel: [w359] -> w348 mode=indexing
          n151 = Bundle By Name(cluster=T14 {"Result"=variant, "CoordinateUse"=FALSE, "CaliperEntry"={"CaliperType"=0, "Points"=[], "Result"={"PointInclude?"=FALSE, "Num_Of_Pts"=0, "Position.X"=0.0, "Position.Y"=0.0, "Angle"=0.0, "Distance"=0.0, "Area"=0.0, "Radius_MAX"=0.0, "Radius2_min"=0.0, "Dev_Residual"=0.0, "P2.X"=0.0, "P2.Y"=0.0, "StepName"="", "Point ID"=0, "StepError?"=FALSE, "ResultDiff?"=FALSE}, "StepName"=""}} ("CoordinateCaliperSetting"), "CaliperEntry"=w358) -> (w359:T14)
          n152 = Unbundle By Name(w358) -> ("StepName"=w360:string)
        }
        n153 = Bundle By Name(cluster=w350, "CaliperSetting"=w348) -> (w349:T22)
        n154 = property on="Caliper Step" class="LstBox (strict)"("Item Names"=w354, "Value"=i32[] [] ("Caliper Step")) -> ()  [unwired: 2 in, 2 out]
      }
      frame "Run Test" {
        w365 = FALSE ("CoordSystemRun?")
        # "若2個都是0則表示為Analysis Step中已經沒有東西"
        n155 = call "IMAQ Copy"("Image Dst"=w399, "Image Src"=w400) -> ("Image Dst Out"=w398:T1)  [unwired: 4 in, 1 out]
        n156 = Unbundle By Name(w393) -> ("AnalysisSetting"=w395:T23[], "ProcessSetting"=w397:T9[])
        n157 = call "Execute_All_Process.vi"("ImageIn"=w398, "ProcessSettingIn"=w397) -> ("error out"=w391:errorcluster, "Image Out"=w394:T1, "Palette Type"=w396:u32)  [unwired: 4 in, 3 out]
        n158 = property on="Vision_Image" class="ImageControl"("Palette Type"=w396) -> ()  [unwired: 2 in, 2 out]
        n159 = call "CoordRunAnalysis.vi"("Refnum in"=w394, "CoordinatteEntry In"=w393, "AnalysisSetting"=w395, "Error In"=w391, "CoordSystemRun?"=w365, "RootPath"=w390) -> ("CoordinatteEntry Out"=w392:T22, "Main Out"=w382:T8[], "Error Out"=w363:errorcluster)  [unwired: 10 in, 1 out]
        n160 = call "[FGV] Analysis_Result_Points.vi"("CoordSystemRun"=w365, "Action"=AnalysisResultPointsAction."ReadAll", "error in (no error)"=w363) -> ("error out"=w376:errorcluster, "Analysis_Point_Result Out"=w373:T29[])  [unwired: 7 in]
        n161 = call "[FGV] Analysis_Result_Points_Overlay.vi"("CoordSystemRun"=w365, "Action"=AnalysisResultPointsAction."ReadAll", "error in (no error)"=w363) -> ("error out"=w371:errorcluster, "Analysis_Point_Result Out"=w362:T29[])  [unwired: 7 in]
        n162 = Unbundle By Name(w392) -> ("AnalysisSetting"=w383:T23[])
        n163 = call "[FGV] CaliperEntry.vi"("CoordSystemRun"=w365, "Action"=Caliper_Entry_FGV_Action."ReadAll", "error in (no error)"=w376) -> ("error out"=w378:errorcluster, "AllCaliperEntries"=w379:T15[])  [unwired: 7 in]
        n164 = call "[FGV] CaliperEntry_Overlay.vi"("CoordSystemRun"=w365, "Action"=Caliper_Entry_FGV_Action."ReadAll", "error in (no error)"=w371) -> ("error out"=w369:errorcluster)  [unwired: 7 in, 1 out]
        n165 = call "CaliperEntrySetToNone.vi"("error in (no error)"=w378, "CaliperEntryList"=w379) -> ("CaliperEntryOut"=w377:T15[])  [unwired: 8 in, 1 out]
        n166 = Array Size(array=w383) -> (size(s)=w388:i32)
        n167 = call "CaliperEntrySetToNone.vi"("error in (no error)"=w369) -> ("CaliperEntryOut"=w368:T15[])  [unwired: 9 in, 1 out]
        n168 = Array Size(array=w382) -> (size(s)=w387:i32)
        n169 = Equal To 0?(x=w388) -> (x = 0?=w386:bool)
        n170 = Equal To 0?(x=w387) -> (x = 0?=w385:bool)
        n171 = call "Run All Caliper Steps.vi"("Analysis_Point_Result"=w373, "CaliperEntryList"=w377) -> ("CaliperEntryOut"=w372:T15[])  [unwired: 9 in]
        n172 = call "Run All Caliper Steps.vi"("Analysis_Point_Result"=w362, "CaliperEntryList"=w368) -> ("CaliperEntryOut"=w364:T15[])  [unwired: 9 in]
        n173 = And(x=w386, y=w385) -> (x .and. y?=w384:bool)
        n174 = call "[FGV] CaliperEntry.vi"("CoordSystemRun"=w365, "Action"=Caliper_Entry_FGV_Action."ReplaceAll", "CaliperEntriesIn"=w372) -> ("error out"=w374:errorcluster)  [unwired: 7 in, 1 out]
        n175 = call "[FGV] CaliperEntry_Overlay.vi"("CoordSystemRun"=w365, "Action"=Caliper_Entry_FGV_Action."ReplaceAll", "CaliperEntriesIn"=w364) -> ()  [unwired: 7 in, 2 out]
        n176 = case shown="False" w384 {
          tunnel: w374 -> [w411 w425]
          tunnel: [w405 w425] -> w389
          tunnel: w383 -> [w410 _]
          tunnel: w382 -> [w409 _]
          tunnel: w373 -> [w402 _]
          tunnel: w364 -> [w403 _]
          frame False {
            (unwired) string[][] [["", "X1", "Y1", "Angle", "", ""]]
            n177 = control-ref of="Vision_Image"() -> (w404:refnum<vi>)
            n178 = control-ref of="Available Points"() -> (w408:refnum<vi>)
            n179 = for {
              tunnel: w409 -> [w423] mode=indexing
              tunnel: w410 -> [w422] mode=indexing
              tunnel: w411 -> [w421]
              shift-right: [w420] -> _
              shift-left: string[][] [] ("Listbox Out") -> [w419]
              tunnel: [w418] -> w406
              tunnel: w408 -> [w417]
              tunnel: w404 -> [w415]
              i -> [w416]
              n180 = call "Update_Analized_CoorOverlay.vi"("Listbox In"=w419, "ROI Entry"=w423, "error in (no error)"=w421, "Available Points In"=w417, "AnalysisResult"=w422, "Image Refnum"=w415) -> ("error out"=w418:errorcluster, "Listbox Out"=w420:string[][])  [unwired: 4 in]
              "Numeric" <- w416
            }
            n181 = for {
              tunnel: w404 -> [w414]
              tunnel: w403 -> [w413] mode=indexing
              tunnel: w402 -> [w412]
              n182 = call "Update_Caliper_Overlay.vi"("Analysis_Point_Result"=w412, "CaliperEntry"=w413, "Image Refnum"=w414) -> ()  [unwired: 9 in]
            }
            n183 = call "UpdateCaliperToCoorResultTable.vi"("Type"=enum16{"TagName", "Value"}."Value", "error in (no error)"=w406, "MCListbox Refnum"=w408) -> ("error out"=w405:errorcluster)  [unwired: 7 in, 1 out]
          }
          frame True {
            n184 = property on="Available Points" class="MCListbox (strict)"("ItemNames"=string[][] [] ("Item Names")) -> ()  [unwired: 2 in, 2 out]
          }
        }
      }
      frame "UpdateOriginList" {
        n185 = Variant To Data(type=T6 {"Row"=0, "Column"=0} ("Cell Position"), Variant=w432) -> (data=w429:T6)  [unwired: 1 in, 1 out]
        n186 = disable-structure shown="Disabled" {
          disable-tunnel: w434 -> [w436 _]
          frame Disabled {
            n187 = control-ref of="Available Points"() -> (w435:refnum<vi>)
            n188 = control-ref of="Vision_Image"() -> (w437:refnum<vi>)
            n189 = call "UpdaeCoorOverlay.vi"("ImageCtl"=w437, "CoordinatePoints"=w435, "Image"=w436) -> ()  [unwired: 8 in, 1 out]
          }
          frame Enabled {
          }
        }
        n190 = control-ref of="Available Points"() -> (w428:refnum<vi>)
        n191 = call "UpdateSelectStatus.vi"("Available Points"=w428, "error in (no error)"=w430, "Available Points Idx"=w429) -> ("error out"=w427:errorcluster)  [unwired: 8 in]
      }
      frame "SetOrigin" {
        n192 = disable-structure shown="Enabled" {
          disable-tunnel: w442 -> [w446 w472]
          disable-tunnel: [w445 w471] -> w441
          disable-tunnel: w439 -> [_ w469]
          disable-tunnel: [_ w468] -> w438
          frame Disabled {
            n193 = property on="Available Points" class="MCListbox (strict)"() -> ("Value"=w444:i32)  [unwired: 2 in, 2 out]
            n194 = Not Equal To 0?(x=w444) -> (x != 0?=w443:bool)
            n195 = case shown="False" w443 {
              tunnel: w446 -> [w447 w449]
              tunnel: [w447 w461] -> w445
              tunnel: w444 -> [_ w454]
              frame False {
              }
              frame True {
                n196 = control-ref of="Available Points"() -> (w450:refnum<vi>)
                n197 = call "SetOrigin.vi"("Available Points in"=w450, "CoordinatteEntry In"=w449) -> ("CoordinatteEntry Out"=w448:T22)  [unwired: 7 in, 2 out]
                n198 = Unbundle By Name(w448) -> ("Coord?"=w462:bool)
                n199 = property on="Available Points" class="MCListbox (strict)"() -> ("ItemNames"=w453:string[][])  [unwired: 2 in, 2 out]
                n200 = Array Size(array=w453) -> (size(s)=w452:i32[])
                n201 = disable-structure shown="Enabled" {
                  disable-tunnel: w462 -> [w464 w467]
                  disable-tunnel: [w463 w467] -> w460
                  frame Disabled {
                    n202 = for {
                      tunnel: w464 -> [w466]
                      tunnel: [w465] -> w463
                      stop <- w465 stop-if-true
                      n203 = Unbundle By Name(w466) -> ("CoordinateUse"=w465)
                    }
                  }
                  frame Enabled {
                  }
                }
                n204 = Index Array(array=w452) -> (element=w451:i32)  [unwired: 1 in]
                n205 = Initialize Array(0 ("element"), w451) -> (w458:i32[])
                n206 = Replace Array Subset(array=w458, new element=1 ("new element/subarray"), index=w454) -> (w456:i32[])
                n207 = property on="Available Points" class="MCListbox (strict)"("ItemSyms"=w456, "Symbols Vis"=TRUE ("Visible Items:Symbols Visible")) -> ()  [unwired: 2 in, 2 out]
                n208 = Bundle By Name(cluster=w448, "Coord?"=w460) -> (w461:T22)
              }
            }
          }
          frame Enabled {
            n209 = control-ref of="Available Points"() -> (w473:refnum<vi>)
            n210 = call "SetOrigin.vi"("Available Points in"=w473, "Error In"=w469, "CoordinatteEntry In"=w472) -> ("Error Out"=w468:errorcluster, "OriginSet?"=→"Origin Set":bool, "CoordinatteEntry Out"=w471:T22)  [unwired: 6 in]
          }
        }
      }
      frame "OriginUpdate" {
        n211 = disable-structure shown="Enabled" {
          disable-tunnel: w478 -> [w483 w503]
          disable-tunnel: w476 -> [_ w500]
          disable-tunnel: [_ w501] -> w475
          disable-tunnel: [_ w502] -> w474
          frame Disabled {
            n212 = Unbundle By Name(w483) -> ("CoordIndex"=w492:i32[])
            n213 = property on="Available Points" class="MCListbox (strict)"() -> ("ItemNames"=w481:string[][])  [unwired: 2 in, 2 out]
            n214 = for {
              tunnel: w492 -> [w495] mode=indexing
              tunnel: [w494] -> w488
              tunnel: [w493] -> w484
              i -> [w493]
              stop <- w494 stop-if-true
              n215 = disable-structure shown="Enabled" {
                disable-tunnel: w495 -> [w497 w498]
                disable-tunnel: [w496 w498] -> w494
                frame Disabled {
                  n216 = Unbundle By Name(w497) -> ("CoordinateUse"=w496)
                }
                frame Enabled {
                }
              }
            }
            n217 = Array Size(array=w481) -> (size(s)=w480:i32[])
            n218 = Index Array(array=w480) -> (element=w479:i32)  [unwired: 1 in]
            n219 = Initialize Array(0 ("element"), w479) -> (w490:i32[])
            n220 = Increment(x=w484) -> (x+1=w482:i32)
            n221 = Select(t=1 ("element"), s=w488, f=0 ("element")) -> (s? t:f=w485:i32)
            n222 = Replace Array Subset(array=w490, new element=w485, index=w482) -> (w489:i32[])
            n223 = property on="Available Points" class="MCListbox (strict)"("ItemSyms"=w489, "Value"=w482) -> ()  [unwired: 2 in, 2 out]
          }
          frame Enabled {
            n224 = control-ref of="Available Points"() -> (w499:refnum<vi>)
            n225 = call "UpdateOriginList.vi"("Available Points"=w499, "error in (no error)"=w500, "CoordinatteEntry In"=w503) -> ("error out"=w501:errorcluster, "CoordinatteEntry Out"=w502:T22)  [unwired: 7 in]
          }
        }
      }
      frame "EditAnalysis" {
        n226 = Unbundle By Name(w518) -> ("Project Name"=w507:string, "AnalysisSetting"=w516:T23[], "ProcessSetting"=w522:T9[])
        n227 = call "IMAQ Copy"("Image Dst"=w508, "Image Src"=w525) -> ("Image Dst Out"=w524:T1)  [unwired: 4 in, 1 out]
        n228 = property on="Analysis Step" class="LstBox (strict)"() -> ("Value"=w520:i32[])  [unwired: 2 in, 2 out]
        n229 = Index Array(array=w520) -> (element=w515:i32)  [unwired: 1 in]
        n230 = Index Array(array=w516, index=w515) -> (element=w517:T23)
        n231 = call "Execute_All_Process.vi"("ImageIn"=w524, "ProcessSettingIn"=w522) -> ("Image Out"=w511:T1, "Palette Type"=w512:u32)  [unwired: 4 in, 4 out]
        n232 = property on="Vision_Image" class="ImageControl"("Palette Type"=w512) -> ()  [unwired: 2 in, 2 out]
        n233 = Unbundle By Name(w517) -> ("Analysis_Type"=w505:enum16{"PatternMatch", "Straight Edge"}, "AnalysisStepName"=w509:string)
        n234 = call "DataEntryTransform.vi"("DataTrasform"=DataTransform."CoordToMain", "CoordSettingIn"=w517) -> ("MainSettingOut"=w519:T11)  [unwired: 7 in, 2 out]
        n235 = control-ref of="Analysis Step"() -> (w523:refnum<vi>)
        n236 = case shown="\"PatternMatch\", Default" w505 {
          tunnel: [w552 w554] -> w510
          tunnel: [w551 w555] -> w514
          tunnel: w511 -> [w550 w558]
          tunnel: w523 -> [w549 w557]
          tunnel: w507 -> [w548 w556]
          tunnel: w519 -> [w547 w553]
          tunnel: w506 -> [w546 _]
          frame "PatternMatch", Default {
            n237 = call "PatternMatch_Setting_UI.vi"("RootPath"=w546, "Type"="Coordinate", "Analysis_Setting In"=w547, "Coord?"=TRUE, "ProjectName"=w548, "LstBox Refnum"=w549, "Vision_Image In"=w550) -> ("Cancel?"=w552:bool, "Analysis_Setting"=w551:T25)  [unwired: 2 in, 1 out]
          }
          frame "Straight Edge" {
            n238 = call "Find Straight Edge.vi"("Analysis_Setting IN"=w553, "ProjectName"=w556, "ROI List IN"=w557, "Vision_Image"=w558) -> ("Cancel?"=w554:bool, "Analysis_Setting"=w555:T27)  [unwired: 5 in, 1 out]
          }
        }
        n239 = case shown="False" w510 {
          tunnel: w518 -> [w542 w543]
          tunnel: [w541 w543] -> w513
          tunnel: w516 -> [w539 _]
          tunnel: w514 -> [w533 _]
          tunnel: w517 -> [w532 _]
          tunnel: w515 -> [w530 _]
          tunnel: w511 -> [w526 _]
          tunnel: w509 -> [w529 _]
          tunnel: w507 -> [w528 _]
          tunnel: w506 -> [w527 _]
          frame False {
            n240 = Bundle(cluster=T8 {"vROIName"="", "vROIContour"={"Contour Type"=0, "ROI Type"=0, "Points"=[]}, "ProcessSetting"=[], "Analysis_Setting"={"PreProcess"=enum."None", "Parameter"=""}} ("ROI Entry"), "Analysis_Setting"=w533) -> (w537:T8)  [unwired: 3 in]
            n241 = call "Execute_Analysis.vi"("Image In"=w526, "ProjectName"=w528, "ROI Entry"=w537, "RootPath"=w527) -> ("Result"=w535:variant)  [unwired: 7 in, 4 out]
            n242 = call "DataEntryTransform.vi"("DataTrasform"=DataTransform."MainToCoord", "AnalysisStepName"=w529, "MainSettingIn"=w533, "CoordSettingIn"=w532) -> ("CoordSettingOut"=w536:T23)  [unwired: 5 in, 2 out]
            n243 = Bundle By Name(cluster=w536, "Step Result"=w535) -> (w531:T23)
            n244 = Replace Array Subset(array=w539, new element=w531, index=w530) -> (w534:T23[])
            n245 = Bundle By Name(cluster=w542, "AnalysisSetting"=w534) -> (w541:T22)
          }
          frame True {
          }
        }
      }
      frame "DeleteAnalysis" {
        n246 = property on="Analysis Step" class="LstBox (strict)"() -> ("Value"=w563:i32[])  [unwired: 2 in, 2 out]
        n247 = control-ref of="Analysis Step"() -> (w562:refnum<vi>)
        n248 = call "DeleteAction.vi"("Error In"=w561, "Analysis List"=w562, "Analysis Step"=w563, "CoordinatteEntry In"=w565) -> ("Error Out"=w560:errorcluster, "CoordinatteEntry Out"=w564:T22)  [unwired: 6 in]
      }
      frame "Init Read Template" {
        n249 = local read "Project Name"() -> (w567:string)
        n250 = call "[FGV]Read Template.vi"("Project Name"=w567, "RootPath"=w570) -> ("error out"=w569:errorcluster)  [unwired: 9 in]
      }
    }
    n251 = call "CoordinateDataEntry.vi"("CoordinateAction"=CoordinateAction."CoordEntryInput", "error in (no error)"=w138, "OneCoordStep Input"=w142) -> ()  [unwired: 7 in, 2 out]
  }
  n252 = call "Imaq Dispose"("Image"=w3) -> ()  [unwired: 5 in, 1 out]
  n253 = call "Imaq Dispose"("Image"=w4) -> ()  [unwired: 5 in, 1 out]
